vi "Sensors_TDMS_write.vi"(0 "TDMS: file name":string="sepiosLOG" caption="default name", 1 "Viewer_enable":bool, 2 "base path":path, 5 "Period [ms]":i64=10, 7 "group name":string="IMU, DepthSensor,CurrentSensor", 9 "channel name(s)":string[](array[string])=["X_Gyro", "Y_Gyro", "Z_Gyro", "X_Accl", "Y_Accl", "Z_Accl", "X_Magn", "Y_Magn", "Z_Magn", "IMU_Temp", "IMU_Barom", "Depth", "Current"], 11 "error in":errorcluster) -> (15 "error out":errorcluster)   [LabVIEW 2013]
uses:
  <vilib>/Platform/TimedLoop/XDataNode/timing_clust.ctl
  <vilib>/Platform/TimedLoop/XDataNode/nitl_modes.ctl
  <vilib>/Platform/TimedLoop/XDataNode/wakeup.ctl
  myRIO/Sensors/IMU/IMU_Data_Type_Def.ctl
  Controls/Estimated Position.ctl
  <vilib>/platform/TimedLoop/XDataNode/XDataNode.xnode
  <vilib>/Platform/TimedLoop/XDataNode/XDNodeRunTimeDep.lvlib
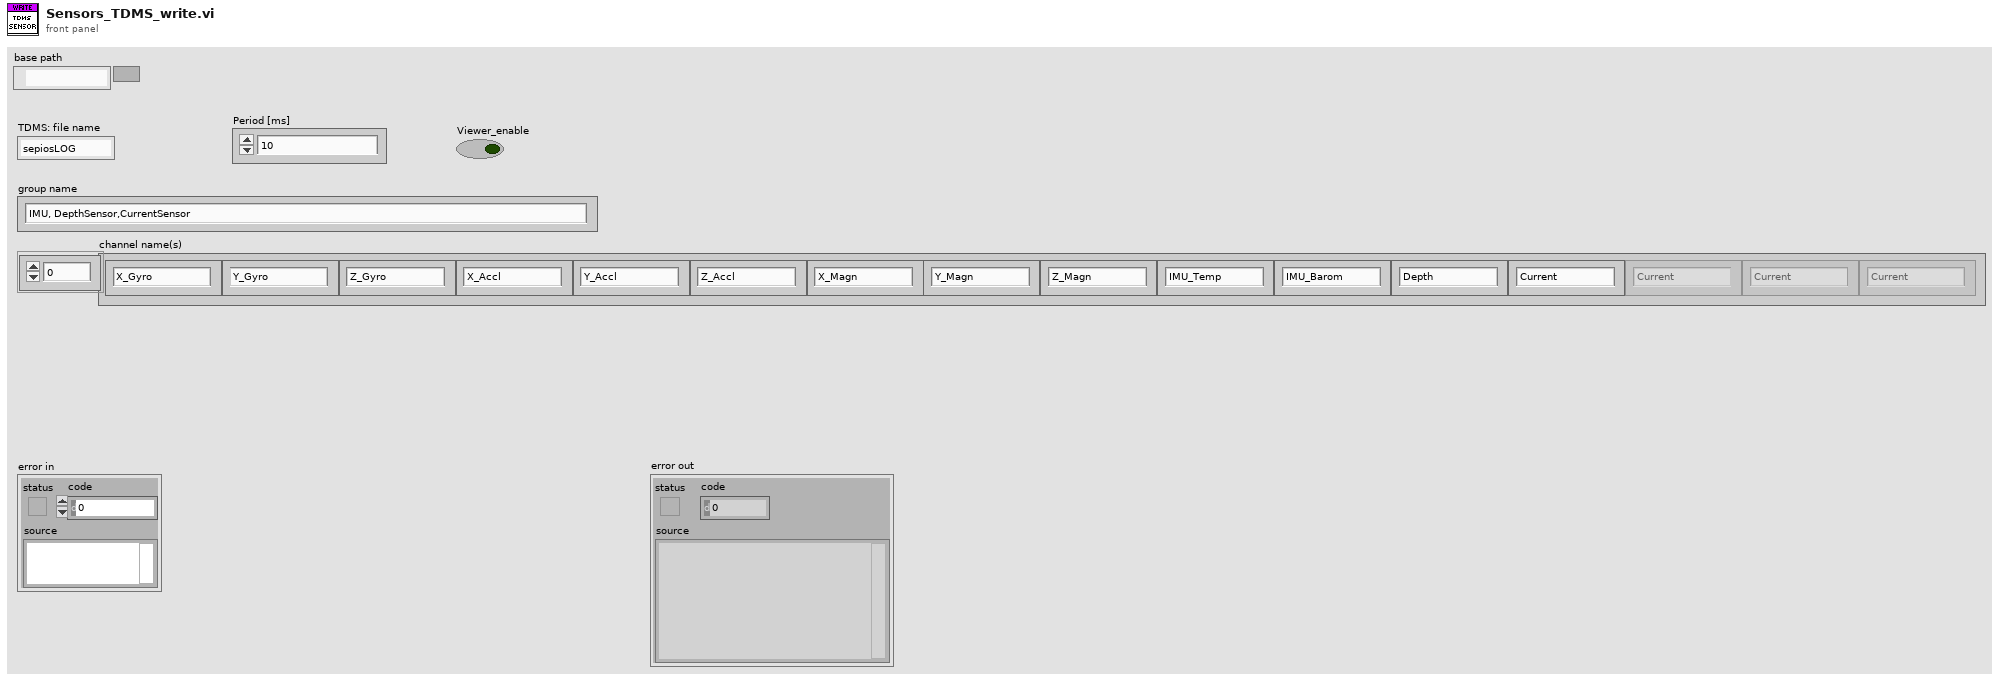
[diagram p1: front panel]
types:
  T1 = enum16{"open", "open or create", "create or replace", "create", "open (read-only)"}
  T2 = typedef "XDNodeRunTimeDep.lvlib/timing_clust.ctl" = cluster{"Expected End [f-1]":u64, "Actual End [f-1]":u64, "Finished Late? [f-1]":bool, "Expected End [i-1]":u64, "Actual End [i-1]":u64, "Finished Late? [i-1]":bool, "Expected Start [i]":u64, "Actual Start [i]":u64, "Expected Start [f]":u64, "Actual Start [f]":u64, "Source Name":string, "Structure Name":string, "Period":i64, "Deadline":i64, "Offset":i64, "Start":i64, "Priority":i32, "Timeout":i32, "Mode":T3, "Wakeup Reason":T4, "Error":errorcluster, "Source Type":string, "Secondary Source Type":string, "Global End Time":u64, "Global Start Time":u64, "Frame Duration":u64, "Iteration Duration":u64, "Assigned CPU":i32, "I/O Scan Engine Mode":u32}
  T3 = typedef "XDNodeRunTimeDep.lvlib/nitl_modes.ctl" = enum32{"No Change", "Process missed periods, maintain original phase", "Discard missed periods, maintain original phase", "Process missed periods, ignore original phase", "Discard missed periods, ignore original phase"}
  T4 = typedef "XDNodeRunTimeDep.lvlib/wakeup.ctl" = enum32{"Normal", "Aborted", "Asynchronous wakeup", "Timing source error", "Timed loop error", "Timeout"}
  T5 = typedef "IMU_Data_Type_Def.ctl" = cluster{timestamp, "X_Gyro_Out":dbl, "Y_Gyro_Out":dbl, "Z_Gyro_Out":dbl, "X_Accl_Out":dbl, "Y_Accl_Out":dbl, "Z_Accl_Out":dbl, "X_Magn_Out":dbl, "Y_Magn_Out":dbl, "Z_Magn_Out":dbl, "Temp_Out":dbl, "Barom_Out":dbl}
  T6 = cluster{"New attitude phi":dbl, "New attitude theta":dbl, "New attitude psi":dbl}
  T7 = typedef "Estimated Position.ctl" = cluster{"X":dbl, "Y":dbl, "Z":dbl, "V_X":dbl, "V_Y":dbl, "V_Z":dbl}
  T8 = cluster{"u_Body":dbl, "v_Body":dbl, "w_Body":dbl, "omega_x_Body":dbl, "omega_z_Body":dbl, "omega_y_Body":dbl}
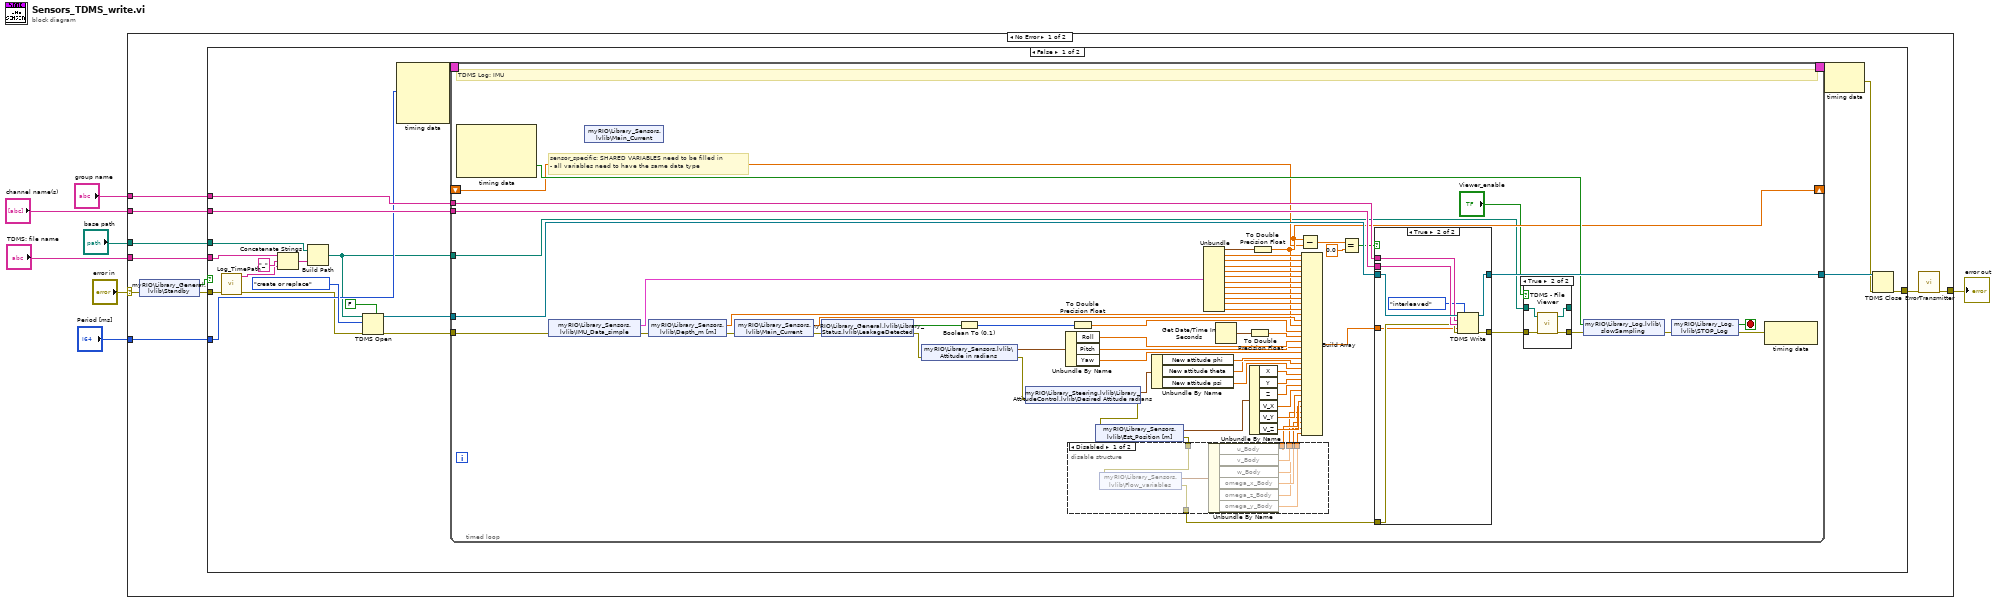
[diagram p0: block diagram]
diagram:
  n1 = case shown="No Error" "error in" {
    selector: "error in" -> [w10 w143]
    tunnel: "group name" -> [w17 _]
    tunnel: "channel name(s)" -> [w16 _]
    tunnel: "Period [ms]" -> [w15 _]
    tunnel: "TDMS: file name" -> [w14 _]
    tunnel: [w8 w143] -> w3
    tunnel: "base path" -> [w13 _]
    frame No Error {
      n2 = shared-variable "myRIO\\Library_General.lvlib\\Standby"(error in=w10) -> (w12:bool, error out=w11:errorcluster)
      n3 = case shown="False" w12 {
        tunnel: w17 -> [w32 _]
        tunnel: w16 -> [w31 _]
        tunnel: w15 -> [w30 _]
        tunnel: w14 -> [w27 _]
        tunnel: w11 -> [w21 w142]
        tunnel: [w22 w142] -> w9
        tunnel: w13 -> [w18 _]
        frame False {
          n4 = call "Log_TimePath.vi"("error in (no error)"=w21) -> ("error out"=w20:errorcluster, "result string"=w19:string)  [unwired: 9 in]
          n5 = Concatenate Strings(w27, "_" ("string"), w19) -> (w28:string)
          n6 = Build Path(base path=w18, name or relative path=w28) -> (appended path=w23:path)
          n7 = TDMS Open(5:FALSE ("create index file? (T)"), 8:w20, 10:T1."create or replace" ("operation (0:open)"), 11:w23) -> (0:w33:errorcluster, 3:w34:refnum<k34>)  [unwired: 3 in]
          n8 = node-c288(w30) -> (w37:T2)  [unwired: 3 in]
          n9 = timed-loop {
            tunnel: w33 -> [w97]
            tunnel: w34 -> [w105]
            tunnel: [w104] -> w29
            tunnel: w31 -> [w103]
            tunnel: w32 -> [w102]
            timing: w37 -> [_]
            timing-out: [_] -> w36
            shift-right: [w80] -> _
            shift-left: _ -> [w79]
            tunnel: w23 -> [w67]
            stop <- w64 stop-if-true
            # "sensor_specific: SHARED VARIABLES need to be filled in\n- all variables need to have the same data type"
            # "TDMS Log: IMU"
            n10 = node-c288() -> (w101:bool)  [unwired: 1 in, 3 out]
            n11 = shared-variable "myRIO\\Library_Sensors.lvlib\\IMU_Data_simple"(error in=w97) -> (w96:T5, error out=w99:errorcluster)
            n12 = shared-variable "myRIO\\Library_Sensors.lvlib\\Main_Current"() -> ()  [unwired: 1 in, 2 out]
            n13 = shared-variable "myRIO\\Library_Sensors.lvlib\\Depth_m [m]"(error in=w99) -> (w82:dbl, error out=w98:errorcluster)
            n14 = shared-variable "myRIO\\Library_Sensors.lvlib\\Main_Current"(error in=w98) -> (w81:dbl, error out=w75:errorcluster)
            n15 = shared-variable "myRIO\\Library_General.lvlib\\Library_Status.lvlib\\LeakageDetected"(error in=w75) -> (w74:bool, error out=w63:errorcluster)
            n16 = shared-variable "myRIO\\Library_Sensors.lvlib\\Attitude in radians"(error in=w63) -> (w62:cluster{"Roll":dbl, "Pitch":dbl, "Yaw":dbl}, error out=w58:errorcluster)
            n17 = Boolean To (0,1)(Boolean=w74) -> (0, 1=w73:i16)
            n18 = shared-variable "myRIO\\Library_Steering.lvlib\\Library_AttitudeControl.lvlib\\Desired Attitude radians"(error in=w58) -> (w57:T6, error out=w54:errorcluster)
            n19 = Unbundle By Name(w62) -> ("Roll"=w61:dbl, "Pitch"=w60:dbl, "Yaw"=w59:dbl)
            n20 = To Double Precision Float(number=w73) -> (double precision float=w72:dbl)
            n21 = shared-variable "myRIO\\Library_Sensors.lvlib\\Est_Position [m]"(error in=w54) -> (w55:T7, error out=w45:errorcluster)
            n22 = disable-structure shown="Disabled" {
              disable-tunnel: w45 -> [w114 w115]
              disable-tunnel: [w113 w115] -> w44
              disable-tunnel: [w111 _] -> w43
              disable-tunnel: [w110 _] -> w42
              disable-tunnel: [w109 _] -> w41
              disable-tunnel: [w108 _] -> w40
              disable-tunnel: [w107 _] -> w39
              disable-tunnel: [w106 _] -> w38
              frame Disabled {
                n23 = shared-variable "myRIO\\Library_Sensors.lvlib\\Flow_variables"(error in=w114) -> (w112:T8, error out=w113:errorcluster)
                n24 = Unbundle By Name(w112) -> ("u_Body"=w111:dbl, "v_Body"=w110:dbl, "w_Body"=w109:dbl, "omega_x_Body"=w108:dbl, "omega_z_Body"=w107:dbl, "omega_y_Body"=w106:dbl)
              }
              frame Enabled {
              }
            }
            n25 = Unbundle By Name(w57) -> ("New attitude phi"=w56:dbl, "New attitude theta"=w53:dbl, "New attitude psi"=w52:dbl)
            n26 = Unbundle(w96) -> (w95:timestamp, "X_Gyro_Out"=w93:dbl, "Y_Gyro_Out"=w92:dbl, "Z_Gyro_Out"=w91:dbl, "X_Accl_Out"=w90:dbl, "Y_Accl_Out"=w89:dbl, "Z_Accl_Out"=w88:dbl, "X_Magn_Out"=w87:dbl, "Y_Magn_Out"=w86:dbl, "Z_Magn_Out"=w85:dbl, "Temp_Out"=w84:dbl, "Barom_Out"=w83:dbl)
            n27 = Get Date/Time In Seconds() -> (seconds since 1Jan1904=w66:timestamp)
            n28 = Unbundle By Name(w55) -> ("X"=w51:dbl, "Y"=w50:dbl, "Z"=w49:dbl, "V_X"=w48:dbl, "V_Y"=w47:dbl, "V_Z"=w46:dbl)
            n29 = To Double Precision Float(number=w66) -> (double precision float=w65:dbl)
            n30 = To Double Precision Float(number=w95) -> (double precision float=w80:dbl)
            n31 = Subtract(x=w80, y=w79) -> (x-y=w78:dbl)
            n32 = Build Array(w93, w92, w91, w90, w89, w88, w87, w86, w85, w84, w83, w82, w81, w80, w72, w65, w61, w60, w59, w56, w53, w52, w51, w50, w49, w48, w47, w46, w43, w42, w41, w40, w39, w38) -> (w94:dbl[])
            n33 = Equal?(x=w78, y=0.0) -> (x = y?=w76:bool)
            n34 = case shown="True" w76 {
              tunnel: w105 -> [w122 w131]
              tunnel: [w122 w130] -> w104
              tunnel: w103 -> [_ w129]
              tunnel: w102 -> [_ w128]
              tunnel: [w123 w127] -> w69
              tunnel: w44 -> [w123 w126]
              tunnel: w94 -> [_ w125]
              frame False {
              }
              frame True {
                n35 = TDMS Write(0:w131, 1:enum16{"decimated", "interleaved"}."interleaved" ("data layout (0:decimated)"), 5:w128, 7:w129, 9:w125, 11:w126) -> (4:w130:refnum<k34>, 15:w127:errorcluster)  [unwired: 2 out]
              }
            }
            n36 = case shown="True" "Viewer_enable" {
              tunnel: w67 -> [w117 w121]
              tunnel: w69 -> [w116 w120]
              tunnel: [w116 w119] -> w68
              tunnel: [w117 w118] -> _
              frame False {
              }
              frame True {
                n37 = call <vilib>:"TDMS - File Viewer.vi"("error in (no error)"=w120, "file path"=w121) -> ("error out"=w119:errorcluster, "file path out"=w118:path)  [unwired: 4 in]
              }
            }
            n38 = shared-variable "myRIO\\Library_Log.lvlib\\slowSampling"(w101, error in=w68) -> (error out=w100:errorcluster)
            n39 = shared-variable "myRIO\\Library_Log.lvlib\\STOP_Log"(error in=w100) -> (w64:bool, error out=w71:errorcluster)
            n40 = node-c288(w71) -> ()  [unwired: 1 out]
          }
          n41 = node-c288(w36) -> (w24:errorcluster)
          n42 = TDMS Close(8:w24, 11:w29) -> (0:w22:errorcluster)  [unwired: 1 out]
        }
        frame True {
        }
      }
      n43 = call "ErrorTransmitter.vi"("Error In"=w9) -> ("Error Out"=w8:errorcluster)  [unwired: 10 in]
    }
    frame Error {
    }
  }
  "error out" <- w3
